vi "Build Nav HTTP.vi"(7 "VolatusAPI":refnum<class "VolatusAPI.lvclass">, 8 "error in (no error)":errorcluster, 11 "HomeHTTPController in":refnum<class "HomeHTTPController.lvclass">) -> (0 "error out":errorcluster, 2 "Nav HTTP":string, 3 "HomeHTTPController out":refnum<class "HomeHTTPController.lvclass">)   [LabVIEW 2020, in "Volatus.lvlib" / "HomeHTTPController.lvclass"]
uses:
  HomeHTTPController.lvclass
  HomeHTTPController.lvclass/HomeHTTPController.ctl
  VolatusAPI/VolatusAPI.lvclass
  HTTP Manager Identity/HTTP Manager Identity.lvclass
  MessageQ/MessageQ.lvclass
  C:/dev/lv20CE/relink/lv-volatus/Volatus/HTTP Manager Identity/HTTP Manager Identity.lvclass
  C:/dev/lv20CE/relink/lv-volatus/Volatus/Identity/Identity.lvclass
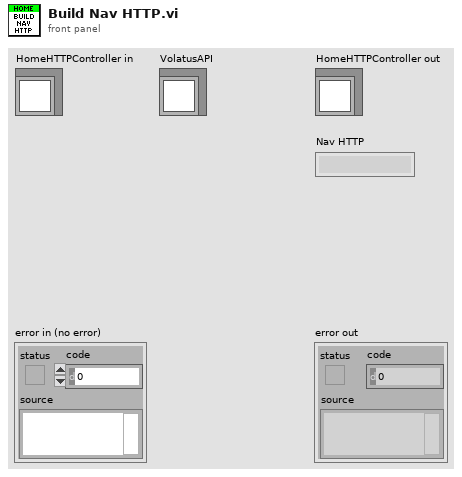
[diagram p1: front panel]
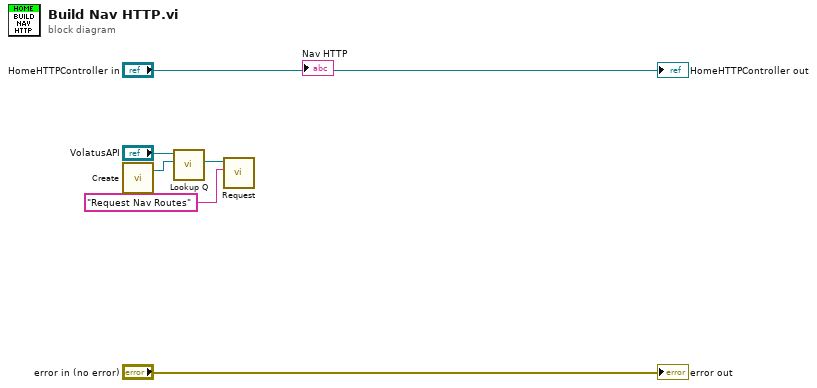
[diagram p0: block diagram]
diagram:
  n1 = call "Create.vi"() -> ("HTTP Manager Identity out"=w3:refnum<class "HTTP Manager Identity.lvclass">)  [unwired: 7 in]
  n2 = call "Lookup Q.vi"("Identity"=w3, "VolatusAPI in"="VolatusAPI") -> ("MessageQ"=w2:refnum<class "MessageQ.lvclass">)  [unwired: 7 in, 2 out]
  n3 = call "Request.vi"("ID"="Request Nav Routes", "MessageQ in"=w2) -> ()  [unwired: 7 in, 3 out]
  "error out" <- "error in (no error)"
  "HomeHTTPController out" <- "HomeHTTPController in"
